vi "Config Sweep.vi"(0 "VISA Resource Name":refnum<visa-resource-name>, 1 "Sweep (0:OFF)":enum16{"OFF", "FREQ", "AMPL", "FREQ & AMPL"}(ring), 2 "Sweep Type (T:LIST)":bool=TRUE, 3 "Sweep Repeat (F:SINGLE)":bool, 4 "Sweep Direction (T:UP)":bool=TRUE, 5 "error in (no error)":errorcluster {"code" format="%.0x"}, 6 "Sweep Trigger (0:IMMEDIATE)":enum16{"IMMEDIATE", "BUS", "EXTERNAL", "KEY"}(ring), 7 "Manual Mode (F:OFF)":bool, 8 "Point Trigger (0:IMMEDIATE)":enum16{"IMMEDIATE", "BUS", "EXTERNAL", "KEY"}(ring), 9 "Manual Point (1)":i32=1, 10 "Trigger In Polarity (T:POS)":bool=TRUE, 12 "Trigger Out Polarity (T:POS)":bool=TRUE) -> (14 "VISA Resource Name Out":refnum<visa-resource-name>, 19 "error out":errorcluster {"code" format="%.0x"})   [LabVIEW 2012, in "Agilent ESG Series.lvlib"]
doc: "This VI is used to set the controls and the parameters associated with frequency and/or power sweeps."
uses:
  <instrlib>/Agilent ESG Series/Agilent ESG Series.lvlib
panel:
  # "ON"
  # "OFF"
  # "UP"
  # "DOWN"
  # "POS"
  # "NEG"
  # "POS"
  # "NEG"
  # "CONT"
  # "SINGLE"
  # "LIST"
  # "STEP"
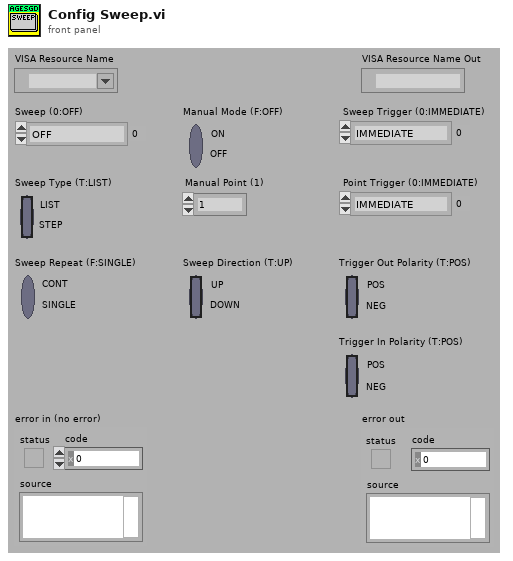
[diagram p1: front panel]
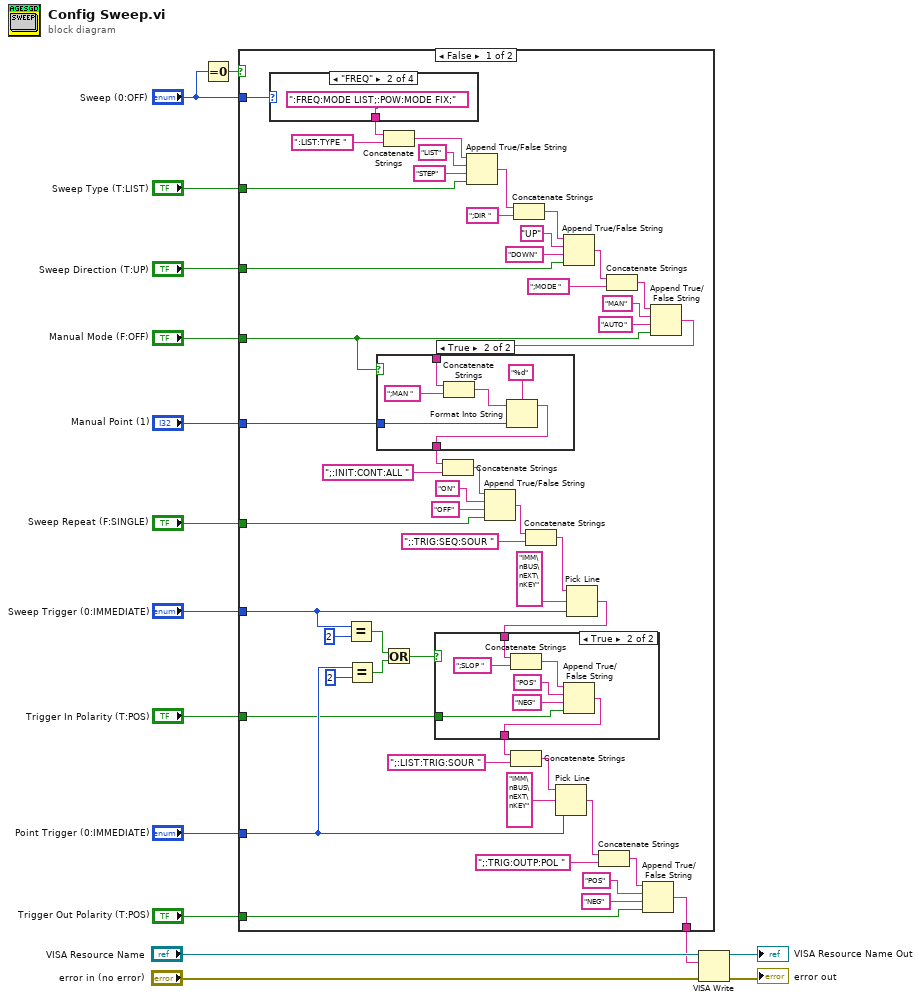
[diagram p0: block diagram]
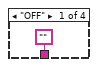
[diagram p4: hidden frame]
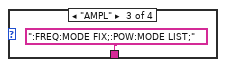
[diagram p5: hidden frame]
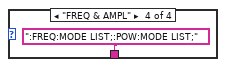
[diagram p6: hidden frame]
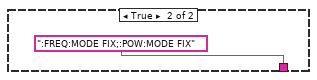
[diagram p7: hidden frame]
diagram:
  n1 = Equal To 0?(x="Sweep (0:OFF)") -> (x = 0?=w2:bool)
  n2 = case shown="False" w2 {
    tunnel: [w17 ":FREQ:MODE FIX;:POW:MODE FIX"] -> w12
    tunnel: "Sweep (0:OFF)" -> [w26 _]
    tunnel: "Sweep Type (T:LIST)" -> [w59 _]
    tunnel: "Sweep Repeat (F:SINGLE)" -> [w58 _]
    tunnel: "Sweep Trigger (0:IMMEDIATE)" -> [w47 _]
    tunnel: "Point Trigger (0:IMMEDIATE)" -> [w43 _]
    tunnel: "Trigger In Polarity (T:POS)" -> [w35 _]
    tunnel: "Trigger Out Polarity (T:POS)" -> [w34 _]
    tunnel: "Sweep Direction (T:UP)" -> [w28 _]
    tunnel: "Manual Point (1)" -> [w25 _]
    tunnel: "Manual Mode (F:OFF)" -> [w18 _]
    frame False {
      n3 = case shown="\"FREQ\"" w26 {
        tunnel: ["" ":FREQ:MODE LIST;:POW:MODE FIX;" ":FREQ:MODE FIX;:POW:MODE LIST;" ":FREQ:MODE LIST;:POW:MODE LIST;"] -> w61
        frame "OFF" {
        }
        frame "FREQ" {
        }
        frame "AMPL" {
        }
        frame "FREQ & AMPL" {
        }
      }
      n4 = Equal?(x=w47, y=i8 2) -> (x = y?=w46:bool)
      n5 = Equal?(x=w43, y=i8 2) -> (x = y?=w42:bool)
      n6 = Concatenate Strings(w61, ":LIST:TYPE ") -> (w60:string)
      n7 = Or(x=w46, y=w42) -> (x .or. y?=w45:bool)
      n8 = Append True/False String(1:w59, 2:"STEP" ("false string"), 3:"LIST" ("true string"), 4:w60) -> (0:w29:string)
      n9 = Concatenate Strings(w29, ";DIR ") -> (w33:string)
      n10 = Append True/False String(1:w28, 2:"DOWN" ("false string"), 3:"UP" ("true string"), 4:w33) -> (0:w27:string)
      n11 = Concatenate Strings(w27, ";MODE " ("string (\"\")")) -> (w22:string)
      n12 = Append True/False String(1:w18, 2:"AUTO" ("false string"), 3:"MAN" ("true string"), 4:w22) -> (0:w23:string)
      n13 = case shown="True" w18 {
        tunnel: [w68 w74] -> w24
        tunnel: w23 -> [w68 w70]
        tunnel: w25 -> [_ w69]
        frame False {
        }
        frame True {
          n14 = Concatenate Strings(w70, ";MAN " ("string (\"\")")) -> (w72:string)
          n15 = Format Into String(format string="%d", initial string=w72, w69) -> (resulting string=w74:string)  [unwired: 1 in, 1 out]
        }
      }
      n16 = Concatenate Strings(w24, ";:INIT:CONT:ALL ") -> (w63:string)
      n17 = Append True/False String(1:w58, 2:"OFF" ("false string"), 3:"ON" ("multi-line string"), 4:w63) -> (0:w55:string)
      n18 = Concatenate Strings(w55, ";:TRIG:SEQ:SOUR ") -> (w53:string)
      n19 = Pick Line(string ("")=w53, multi-line string="IMM\nBUS\nEXT\nKEY", line index=w47) -> (output string=w49:string)
      n20 = case shown="True" w45 {
        tunnel: w49 -> [w75 w78]
        tunnel: [w75 w77] -> w41
        tunnel: w35 -> [_ w76]
        frame False {
        }
        frame True {
          n21 = Concatenate Strings(w78, ";SLOP ") -> (w82:string)
          n22 = Append True/False String(1:w76, 2:"NEG" ("false string"), 3:"POS" ("true string"), 4:w82) -> (0:w77:string)
        }
      }
      n23 = Concatenate Strings(w41, ";:LIST:TRIG:SOUR ") -> (w50:string)
      n24 = Pick Line(string ("")=w50, multi-line string="IMM\nBUS\nEXT\nKEY", line index=w43) -> (output string=w36:string)
      n25 = Concatenate Strings(w36, ";:TRIG:OUTP:POL ") -> (w40:string)
      n26 = Append True/False String(1:w34, 2:"NEG" ("false string"), 3:"POS" ("true string"), 4:w40) -> (0:w17:string)
    }
    frame True {
    }
  }
  n27 = VISA Write(VISA resource name="VISA Resource Name", write buffer=w12, error in (no error)="error in (no error)") -> (VISA resource name out=→"VISA Resource Name Out":refnum<visa-resource-name>, error out=→"error out":errorcluster)  [unwired: 1 out]
